vi "test 2btn dialog with tmo.vi"() -> ()   [LabVIEW 2017]
panel:
  out "T button?":bool
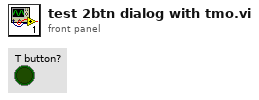
[diagram p1: front panel]
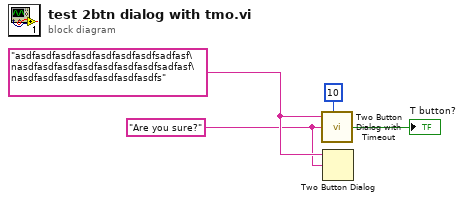
[diagram p0: block diagram]
diagram:
  w1 = "Are you sure?" ("T button name (\"OK\")")
  w3 = "asdfasdfasdfasdfasdfasdfasdfsadfasf\nasdfasdfasdfasdfasdfasdfasdfsadfasf\nasdfasdfasdfasdfasdfasdfasdfs" ("Text")
  n1 = call "Two Button Dialog with Timeout.vi"("message"=w3, "T Timeout(-1 s)"=10, "T button name (\"OK\")"=w1) -> ("T button?"=→"T button?":bool)  [unwired: 2 in]
  n2 = Two Button Dialog(message=w3, 2:w1) -> ()  [unwired: 1 in, 1 out]
